vi "Query with Scalar Integer Result.vi"(8 "error in (no error)":errorcluster, 10 "Query string":string, 11 "sqlite3 in":refnum<class "sqlite3.lvclass">) -> (0 "error out":errorcluster, 2 "Result":i32, 3 "sqlite3 out":refnum<class "sqlite3.lvclass">)   [LabVIEW 2020, in "sqlite3.lvlib" / "sqlite3.lvclass"]
uses:
  sqlite3.lvclass
  sqlite3.lvclass/sqlite3.ctl
  bf923d74-df14-4e6c-8741-a0a90a419c47.vi
  sqlite/VIs/open v2.vi
  sqlite/VIs/close v2.vi
  sqlite/VIs/prepare v2.vi
  sqlite/VIs/step.vi
  sqlite/VIs/column count.vi
  db layer/compound/Resolve Result Type.vi
  bf923d74-df14-4e6c-8741-a0a90a419c47.vi/0244caef-bc9a-4150-a8ac-bf3d364b181c.vi
  bf923d74-df14-4e6c-8741-a0a90a419c47.vi/5568208c-18c9-421a-afbc-e39208249946.vi
  sqlite/VIs/finalize.vi
  sqlite/subvi/Error Converter (ErrCode or Status).vi
  sqlite/VIs/column type.vi
  sqlite/VIs/column int.vi
  bf923d74-df14-4e6c-8741-a0a90a419c47.vi/0244caef-bc9a-4150-a8ac-bf3d364b181c.vi/e2175d81-4f24-490a-8437-0be1725fd2b2.vi
  bf923d74-df14-4e6c-8741-a0a90a419c47.vi/5568208c-18c9-421a-afbc-e39208249946.vi/3e9b31b0-cad7-485d-bd7f-0f335752ecdb.vi
  sqlite/VIs/errstr.vi
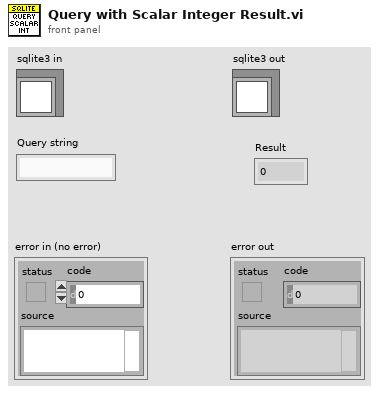
[diagram p1: front panel]
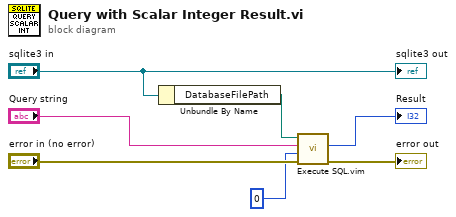
[diagram p0: block diagram]
diagram:
  n1 = Unbundle By Name("sqlite3 in") -> ("DatabaseFilePath"=w5:path)
  n2 = call "Execute SQL.vim"("error in (no error)"="error in (no error)", "desired return type(none)"=0 ("Result"), "sql (string)"="Query string", "database in"=w5) -> ("error out"=→"error out":errorcluster, "Query Result"=→"Result":i32)  [unwired: 6 in]
  "sqlite3 out" <- "sqlite3 in"
